vi "E55555.vi"(8 "error in (no error)":errorcluster, 11 "Data":i32[](array[numeric])) -> (0 "error out":errorcluster)   [LabVIEW 2022 SP3, in "Demo.lvlib" / "E55555.lvclass"]
uses:
  E55555.lvclass
  C:/Users/jakub/repos/gh/lv-error/Source/Error/Error/Error.lvclass
  E55555.lvclass/E55555.ctl
  Error/Error/Error.lvclass
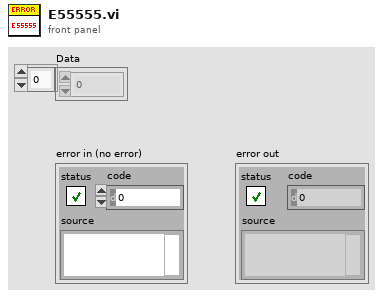
[diagram p1: front panel]
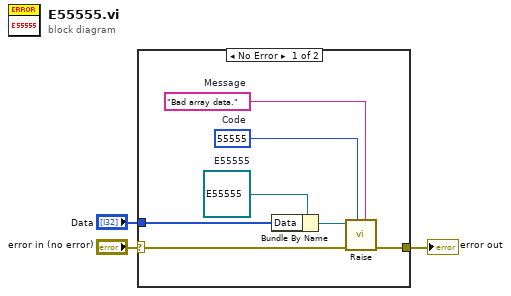
[diagram p0: block diagram]
diagram:
  n1 = case shown="No Error" "error in (no error)" {
    selector: "error in (no error)" -> [w10 w11]
    tunnel: [w8 w11] -> w2
    tunnel: "Data" -> [w6 _]
    frame No Error {
      w4 = "Bad array data."  # Message
      w5 = 55555  # Code
      w9 = refnum<class "E55555.lvclass"> refnum  # E55555
      n2 = Bundle By Name(cluster=w9, "Data"=w6) -> (w7:refnum<class "E55555.lvclass">)
      n3 = call "Raise.vi"("Message"=w4, "Code"=w5, "error in (no error)"=w10, "Error in"=w7) -> ("error out"=w8:errorcluster)  [unwired: 6 in, 1 out]
    }
    frame Error {
    }
  }
  "error out" <- w2
